vi "Fill.vi"(0 "GEA2 Reference In":refnum<k24>, 5 "Standalone?":bool, 7 "Acquisition Rate (Hz)":dbl=10.0 format="%0.2f", 9 "ERDs to Write":string[](array[string])=["01F11D0C010000000200000000000000", "01F11D0C000000000000000000000000", "01F10C0102", "01F10C0106", "01F1080100", "01F1050100", "01F1090100", "0130050101", "01F11D0C010000000100000000000000", "01F11D0C000000000000000000000000"], 11 "Error In":errorcluster, 12 "Expected Hot ON Time (s)":dbl, 13 "Expected Cold ON Time (s)":dbl, 14 "Allowable ON Time Error (s)":dbl) -> (4 "GEA2 Reference Out":refnum<k24>, 6 "Pass/Fail?":bool, 8 "Report Text":string, 10 "Valve ON Time":dbl[][](array[numeric]), 15 "Error Out":errorcluster)   [LabVIEW 2016, in "2015 VA Washer.lvlib"]
doc: "This VI performs a test to ensure the washer MC fills the tub with the appropriate amount of hot and cold water."
uses:
  Projects/2015 VA Washer.lvlib
  C:/Automation/DLLs/PC Dot Net/GeaCommunication.dll
  Common/LabVIEW GEA2 Toolkit/LabVIEW_GEA2_Toolkit.lvlibp/type defs/Data In.ctl
  <vilib>/DAQmx/write.llb/DAQmx Write (Digital 1D Bool NChan 1Samp 1Line).vi
  <vilib>/DAQmx/read.llb/DAQmx Read (Digital 1D Wfm NChan NSamp).vi
  <vilib>/DAQmx/create/channels.llb/DAQmx Create Channel (DI-Digital Input).vi
  <vilib>/DAQmx/create/channels.llb/DAQmx Create Channel (DO-Digital Output).vi
  <vilib>/DAQmx/miscellaneous.llb/DAQmx Fill In Error Info.vi
  <vilib>/DAQmx/configure/timing.llb/DAQmx Timing (Sample Clock).vi
  Common/LabVIEW GEA2 Toolkit/LabVIEW_GEA2_Toolkit.lvlibp
panel:
  out "Lower Limits":dbl[][](array[numeric])
  out "Upper Limits":dbl[][](array[numeric])
  in  "9481_1 Lines":tag="9481_1/port0/line0:9481_1/port0/line3"
  in  "Hot/Cold Valve Lines":tag="9435_1/port0/line3, 9435_2/port0/line0"
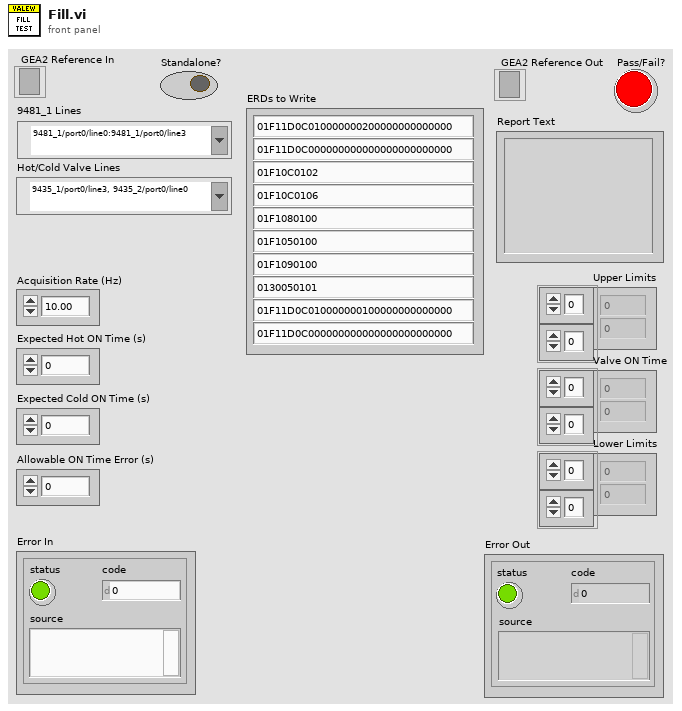
[diagram p1: front panel]
types:
  T1 = typedef "LabVIEW_GEA2_Toolkit.lvlibp/Data In.ctl" = cluster{"Source":u8, "Destination":u8, "Command":u8, "Message":string}
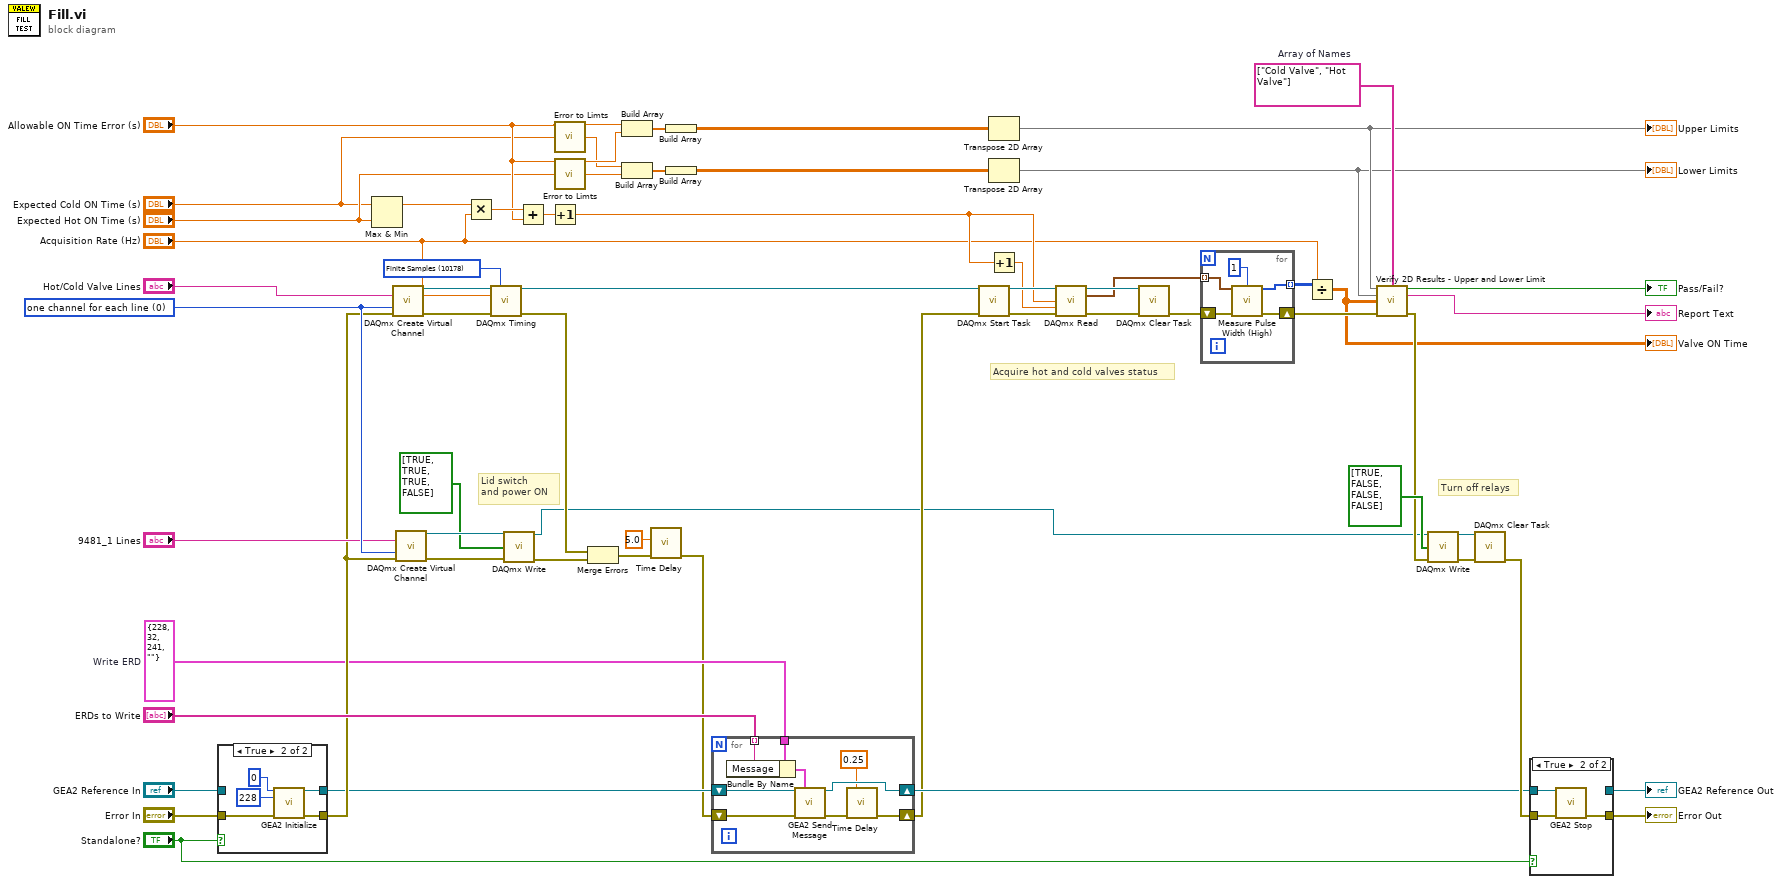
[diagram p0: block diagram]
diagram:
  w6 = T1 {"Source"=228, "Destination"=32, "Command"=241, "Message"=""}  # Write ERD
  w16 = string[] ["Cold Valve", "Hot Valve"]  # Array of Names
  w47 = 0 items=["one channel for each line", "one channel for all lines"] ("line grouping")
  w53 = 10178 items=["Finite Samples"=10178, "Continuous Samples"=10123, "Hardware Timed Single Point"=12522] ("sample mode")
  # "Turn off relays"
  # "Acquire hot and cold valves status"
  # "Lid switch\nand power ON"
  n1 = case shown="True" "Standalone?" {
    tunnel: "Error In" -> [w65 w68]
    tunnel: [w64 w67] -> w7
    tunnel: [w65 w66] -> w40
    tunnel: "GEA2 Reference In" -> [w64 _]
    frame False {
    }
    frame True {
      n2 = call "GEA2 Initialize.vi"("Board Index"=0, "Source Address"=u8 228, "error in"=w68) -> ("GEA2 Reference Out"=w67:refnum<k24>, "error out"=w66:errorcluster)  [unwired: 10 in, 1 out]
    }
  }
  n3 = Max & Min(x="Expected Cold ON Time (s)", y="Expected Hot ON Time (s)") -> (max(x,y)=w52:dbl)  [unwired: 1 out]
  n4 = call-poly <vilib>:"DAQmx Create Virtual Channel.vi"("lines"="Hot/Cold Valve Lines", "line grouping"=w47, "error in"=w40) -> ("task out"=w56:refnum<k21>, "error out"=w55:errorcluster)  [unwired: 11 in]
  n5 = call-poly <vilib>:"DAQmx Create Virtual Channel.vi"("lines"="9481_1 Lines", "line grouping"=w47, "error in"=w40) -> ("task out"=w63:refnum<k21>, "error out"=w45:errorcluster)  [unwired: 11 in]
  n6 = Multiply(x=w52, y="Acquisition Rate (Hz)") -> (x*y=w36:dbl)
  n7 = call-poly <vilib>:"DAQmx Timing.vi"("task/channels in"=w56, "sample mode"=w53, "rate"="Acquisition Rate (Hz)", "error in"=w55) -> ("task out"=w54:refnum<k21>, "error out"=w38:errorcluster)  [unwired: 10 in]
  n8 = call-poly <vilib>:"DAQmx Write.vi"("task/channels in"=w63, "data"=bool[] [TRUE, TRUE, TRUE, FALSE], "error in"=w45) -> ("task out"=w4:refnum<k21>, "error out"=w39:errorcluster)  [unwired: 10 in, 1 out]
  n9 = Add(x=w36, y="Allowable ON Time Error (s)") -> (x+y=w35:dbl)
  n10 = Increment(x=w35) -> (x+1=w34:dbl)
  n11 = call "Error to Limts.vi"("Error"="Allowable ON Time Error (s)", "Value"="Expected Cold ON Time (s)") -> ("Upper Limit"=w31:dbl, "Lower Limit"=w29:dbl)  [unwired: 12 in]
  n12 = call "Error to Limts.vi"("Error"="Allowable ON Time Error (s)", "Value"="Expected Hot ON Time (s)") -> ("Upper Limit"=w30:dbl, "Lower Limit"=w28:dbl)  [unwired: 12 in]
  n13 = Merge Errors(w38, w39) -> (w3:errorcluster)
  n14 = Build Array(w31, w30) -> (w21:dbl[])
  n15 = Build Array(w29, w28) -> (w20:dbl[])
  n16 = call "Time Delay"("error in (no error)"=w3, "Delay Time (s)"=5.0) -> ("error out"=w1:errorcluster)  [unwired: 9 in]
  n17 = Build Array(w21) -> (w19:dbl[][])
  n18 = Build Array(w20) -> (w18:dbl[][])
  n19 = for {
    shift-right: [w72] -> w5
    shift-left: w1 -> [w71]
    shift-right: [w79] -> w8
    shift-left: w7 -> [w78]
    tunnel: w6 -> [w76]
    tunnel: "ERDs to Write" -> [w75] mode=indexing
    n20 = Bundle By Name(cluster=w76, "Message"=w75) -> (w77:T1)
    n21 = call "GEA2 Send Message.vi"("GEA2 Reference In"=w78, "Input Data"=w77, "Error In"=w71) -> ("GEA2 Reference Out"=w79:refnum<k24>, "Error Out"=w73:errorcluster)  [unwired: 11 in]
    n22 = call "Time Delay"("error in (no error)"=w73, "Delay Time (s)"=0.25) -> ("error out"=w72:errorcluster)  [unwired: 9 in]
  }
  n23 = call <vilib>:"DAQmx Start Task.vi"("task/channels in"=w54, "error in"=w5) -> ("task out"=w57:refnum<k21>, "error out"=w58:errorcluster)  [unwired: 12 in]
  n24 = Transpose 2D Array(2D array=w19) -> (transposed array=w11:dbl[][])
  "Upper Limits" <- w11
  n25 = Transpose 2D Array(2D array=w18) -> (transposed array=w10:dbl[][])
  "Lower Limits" <- w10
  n26 = Increment(x=w34) -> (x+1=w33:dbl)
  n27 = call-poly <vilib>:"DAQmx Read.vi"("task/channels in"=w57, "number of samples per channel"=w34, "timeout"=w33, "error in"=w58) -> ("task out"=w60:refnum<k21>, "data"=w43:digitalwaveform[], "error out"=w59:errorcluster)  [unwired: 9 in]
  n28 = call <vilib>:"DAQmx Clear Task.vi"("task in"=w60, "error in"=w59) -> ("error out"=w46:errorcluster)  [unwired: 13 in]
  n29 = for {
    tunnel: w43 -> [w84] mode=indexing
    shift-right: [w82] -> w24
    shift-left: w46 -> [w83]
    tunnel: [w80] -> w17 mode=indexing
    n30 = call "Measure Pulse Width (High).vi"("Input Waveform"=w84, "Minimum Pulse Width"=1, "Error In"=w83) -> ("High Iterations"=w80:i32[], "Error Out"=w82:errorcluster)  [unwired: 11 in]
  }
  n31 = Divide(x=w17, y="Acquisition Rate (Hz)") -> (x/y=w9:dbl[][])
  "Valve ON Time" <- w9
  n32 = call "Verify 2D Results - Upper and Lower Limit.vi"("Upper Limits"=w11, "Array of Names"=w16, "Lower Limits"=w10, "Results"=w9, "Error In"=w24) -> ("Pass/Fail?"=→"Pass/Fail?":bool, "Report Text"=→"Report Text":string, "Error Out"=w25:errorcluster)  [unwired: 7 in, 1 out]
  n33 = call-poly <vilib>:"DAQmx Write.vi"("task/channels in"=w4, "data"=bool[] [TRUE, FALSE, FALSE, FALSE], "error in"=w25) -> ("task out"=w13:refnum<k21>, "error out"=w14:errorcluster)  [unwired: 10 in, 1 out]
  n34 = call <vilib>:"DAQmx Clear Task.vi"("task in"=w13, "error in"=w14) -> ("error out"=w12:errorcluster)  [unwired: 13 in]
  n35 = case shown="True" "Standalone?" {
    tunnel: w12 -> [w86 w89]
    tunnel: [w86 w88] -> w50
    tunnel: w8 -> [w85 w87]
    tunnel: [w85 _] -> w42
    frame False {
    }
    frame True {
      n36 = call "GEA2 Stop.vi"("GEA2 Reference In"=w87, "Error In"=w89) -> ("Error Out"=w88:errorcluster)  [unwired: 13 in]
    }
  }
  "Error Out" <- w50
  "GEA2 Reference Out" <- w42
